vi "Find Level.vi"(11 "Card":T2[](array[typedef])) -> (3 "Level":T1)   [LabVIEW 2023]
uses:
  ENUM_Card.ctl
  ENUM_Level.ctl
  <vilib>/Utility/miscctls.llb/LVMapReplaceAction.ctl
panel:
  out "sorted array":cluster{"Numeric":i32, "Card":T2}[](array[cluster])
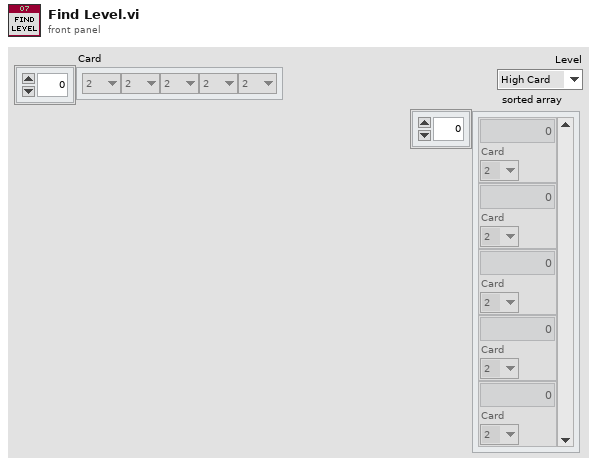
[diagram p1: front panel]
types:
  T1 = typedef "ENUM_Level.ctl" = enum16{"High Card", "One Pair", "Two Pair", "3 of a Kind", "Full House", "4 of a Kind", "5 of a Kind"}
  T2 = typedef "ENUM_Card.ctl" = enum16{"2", "3", "4", "5", "6", "7", "8", "9", "T", "J", "Q", "K", "A"}
  T3 = typedef "LVMapReplaceAction.ctl" = enum32{"Modify Entry only if found", "Add or Modify Entry", "Delete Entry"}
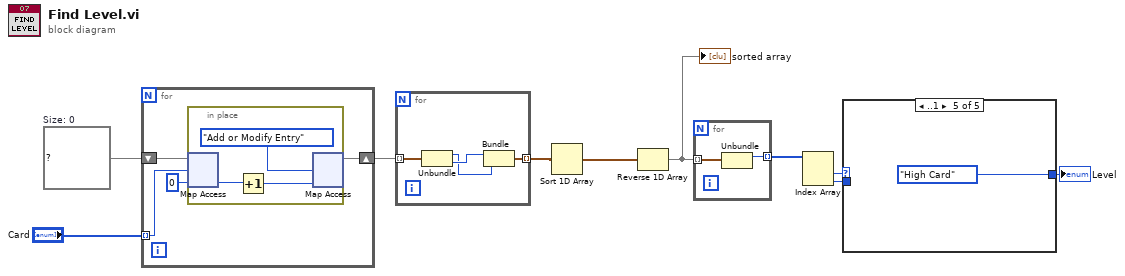
[diagram p0: block diagram]
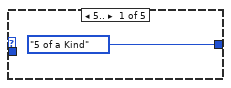
[diagram p2: hidden frame]
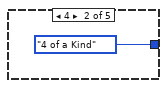
[diagram p3: hidden frame]
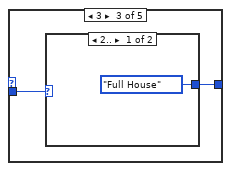
[diagram p4: hidden frame]
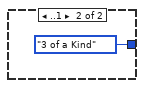
[diagram p5: hidden frame]
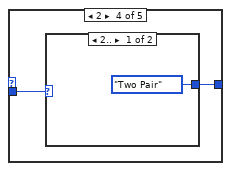
[diagram p6: hidden frame]
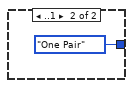
[diagram p7: hidden frame]
diagram:
  w9 = map{T2, i32} {}  # Size: 0
  n1 = for {
    tunnel: "Card" -> [w12] mode=indexing
    shift-right: [w13] -> w8
    shift-left: w9 -> [w14]
    n2 = in-place {
      n3 = in-place-map #1(w14, w12, 0) -> (w16:i32)  [unwired: 1 out]
      n4 = Increment(x=w16) -> (x+1=w15:i32)
      n5 = in-place-map #1(w15, LVMapReplaceAction."Add or Modify Entry" ("action")) -> (w13:map{T2, i32})  [unwired: 2 out]
    }
  }
  n6 = for {
    tunnel: w8 -> [w21] mode=indexing
    tunnel: [w18] -> w7 mode=indexing
    n7 = Unbundle(w21) -> ("Card"=w19:T2, w20:i32)
    n8 = Bundle(w20, "Card"=w19) -> (w18:cluster{i32, "Card":T2})  [unwired: 1 in]
  }
  n9 = Sort 1D Array(array=w7) -> (sorted array=w6:cluster{i32, "Card":T2}[])
  n10 = Reverse 1D Array(array=w6) -> (reversed array=w4:cluster{i32, "Card":T2}[])
  "sorted array" <- w4
  n11 = for {
    tunnel: w4 -> [w23] mode=indexing
    tunnel: [w22] -> w5 mode=indexing
    n12 = Unbundle(w23) -> (w22:i32)  [unwired: 1 out]
  }
  n13 = Index Array(array=w5) -> (element #1=w3:i32, element #2=w1:i32)  [unwired: 2 in]
  n14 = case shown="..1" w3 {
    tunnel: [ENUM_Level."5 of a Kind" ("rank") ENUM_Level."4 of a Kind" ("rank") w27 w31 ENUM_Level."High Card" ("rank")] -> w2
    tunnel: w1 -> [_ _ w26 w30 _]
    frame 5.. {
    }
    frame 4 {
    }
    frame 3 {
      n15 = case shown="2.." w26 {
        tunnel: [ENUM_Level."Full House" ("rank") ENUM_Level."3 of a Kind" ("rank")] -> w27
        frame 2.. {
        }
        frame ..1 {
        }
      }
    }
    frame 2 {
      n16 = case shown="2.." w30 {
        tunnel: [ENUM_Level."Two Pair" ("rank") ENUM_Level."One Pair" ("rank")] -> w31
        frame 2.. {
        }
        frame ..1 {
        }
      }
    }
    frame ..1 {
    }
  }
  "Level" <- w2
